vi "Scan Piezo.vi"(8 "error in (no error)":errorcluster, 9 "notifier out 2":refnum<notifier>, 10 "data":T1, 11 "Hardware Resources In":T2={"Piezo Serial Number"=41848555, "MG17Piezo"=refnum, "Setpoint (um)"=0.0}) -> (0 "error out":errorcluster, 3 "Hardware Resources Out":T2={"Piezo Serial Number"=41848555, "MG17Piezo"=refnum, "Setpoint (um)"=0.0})   [LabVIEW 2013, in "Piezo.lvlib"]
uses:
  Desktop/Simon Labview/Piezo.lvlib
  <vilib>/Platform/TimedLoop/XDataNode/wakeup.ctl
  <vilib>/Platform/TimedLoop/XDataNode/XDNodeRunTimeDep.lvlib
  <vilib>/Platform/TimedLoop/XDataNode/nitl_modes.ctl
  <vilib>/Platform/TimedLoop/XDataNode/timing_clust.ctl
  <vilib>/Platform/TimedLoop/XDataNode/XDataNode.xnode
  <vilib>/Platform/TimedLoop/scheduler/LVUserAPI/_suppVIs/Create_1kHz_TSource.vi
  Piezo State.ctl
  Hardware Configuration.ctl
  Piezo display.ctl
panel:
  in  "Scan Over":bool
  in  "Set Point":dbl
  out "Total Execution Time (s)":dbl
  out "Lag!!":bool
  in  "?":bool
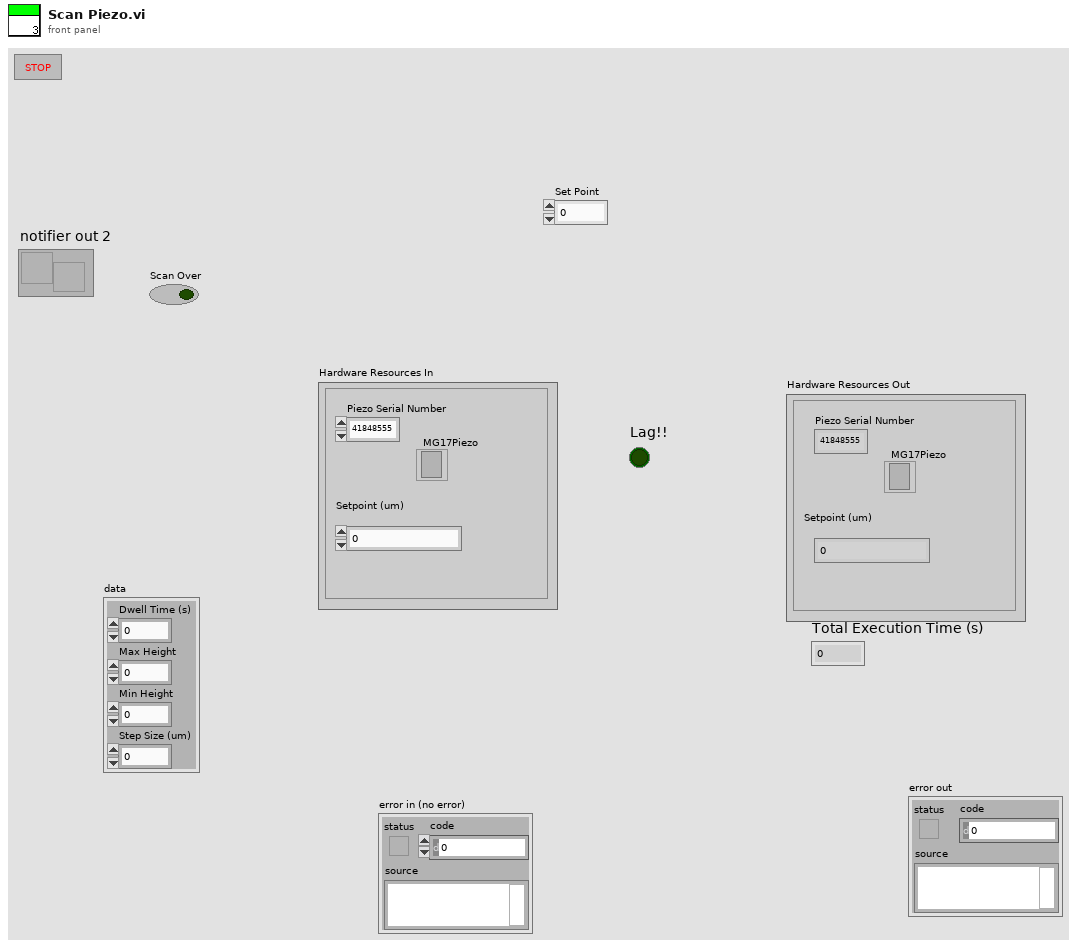
[diagram p1: front panel]
types:
  T1 = cluster{"Dwell Time (s)":dbl, "Max Height":dbl, "Min Height":dbl, "Step Size (um)":dbl}
  T2 = typedef "Piezo.lvlib/Hardware Configuration.ctl" = cluster{"Piezo Serial Number":i32, "MG17Piezo":refnum<k7>, "Setpoint (um)":sgl}
  T3 = typedef "XDNodeRunTimeDep.lvlib/timing_clust.ctl" = cluster{"Expected End [f-1]":u64, "Actual End [f-1]":u64, "Finished Late? [f-1]":bool, "Expected End [i-1]":u64, "Actual End [i-1]":u64, "Finished Late? [i-1]":bool, "Expected Start [i]":u64, "Actual Start [i]":u64, "Expected Start [f]":u64, "Actual Start [f]":u64, "Source Name":string, "Structure Name":string, "Period":i64, "Deadline":i64, "Offset":i64, "Start":i64, "Priority":i32, "Timeout":i32, "Mode":T4, "Wakeup Reason":T5, "Error":errorcluster, "Source Type":string, "Secondary Source Type":string, "Global End Time":u64, "Global Start Time":u64, "Frame Duration":u64, "Iteration Duration":u64, "Assigned CPU":i32, "I/O Scan Engine Mode":u32}
  T4 = typedef "XDNodeRunTimeDep.lvlib/nitl_modes.ctl" = enum32{"No Change", "Process missed periods, maintain original phase", "Discard missed periods, maintain original phase", "Process missed periods, ignore original phase", "Discard missed periods, ignore original phase"}
  T5 = typedef "XDNodeRunTimeDep.lvlib/wakeup.ctl" = enum32{"Normal", "Aborted", "Asynchronous wakeup", "Timing source error", "Timed loop error", "Timeout"}
  T6 = typedef "Piezo.lvlib/Piezo State.ctl" = enum16{"Idle", "Acquiring"}
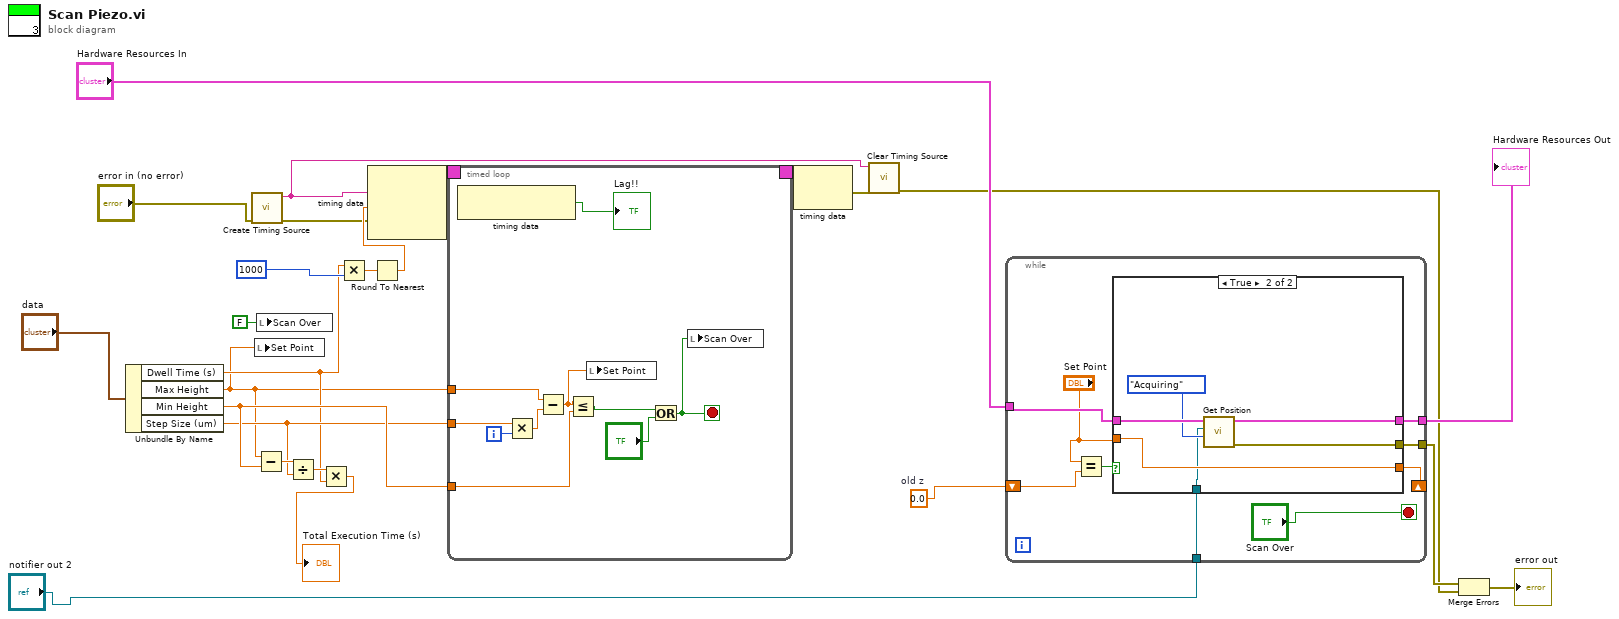
[diagram p0: block diagram]
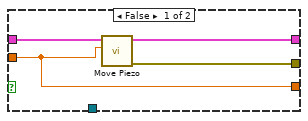
[diagram p2: hidden frame]
diagram:
  w14 = sgl 0.0  # old z
  n1 = Unbundle By Name("data") -> ("Dwell Time (s)"=w16:dbl, "Max Height"=w3:dbl, "Min Height"=w20:dbl, "Step Size (um)"=w18:dbl)
  n2 = call-poly <vilib>:"Create Timing Source.vi"("error in (no error)"="error in (no error)") -> ("error out"=w7:errorcluster, "name (out)"=w6:string)  [unwired: 9 in]
  n3 = local write "Set Point"(w3) -> ()
  n4 = Subtract(x=w3, y=w20) -> (x-y=w19:dbl)
  n5 = local write "Scan Over"(FALSE ("Scan Over")) -> ()
  n6 = Divide(x=w19, y=w18) -> (x/y=w17:dbl)
  n7 = Multiply(x=w17, y=w16) -> (x*y=→"Total Execution Time (s)":dbl)
  n8 = Multiply(x=w16, y=1000) -> (x*y=w22:dbl)
  n9 = Round To Nearest(number=w22) -> (nearest integer value=w21:dbl)
  n10 = node-c288(w6, w21, w7) -> (w25:T3)
  n11 = timed-loop {
    timing: w25 -> [_]
    timing-out: [_] -> w24
    tunnel: w18 -> [w32]
    tunnel: w20 -> [w27]
    tunnel: w3 -> [w30]
    i -> [w31]
    stop <- w29 stop-if-true
    n12 = node-c288() -> (→"Lag!!":bool)  [unwired: 1 in]
    n13 = Multiply(x=w32, y=w31) -> (x*y=w33:dbl)
    n14 = Subtract(x=w30, y=w33) -> (x-y=w26:dbl)
    n15 = Less Or Equal?(x=w26, y=w27) -> (x <= y?=w28:bool)
    n16 = local write "Set Point"(w26) -> ()
    n17 = Or(x=w28, y="?") -> (x .or. y?=w29:bool)
    n18 = local write "Scan Over"(w29) -> ()
  }
  n19 = node-c288(w24) -> (w5:errorcluster)
  n20 = call <vilib>:"Clear Timing Source.vi"("error in (no error)"=w5, "name"=w6) -> ("error out"=w4:errorcluster)  [unwired: 8 in, 1 out]
  n21 = while {
    tunnel: [w47] -> w13
    tunnel: [w46] -> w10
    tunnel: "notifier out 2" -> [w44]
    shift-right: [w43] -> _
    shift-left: w14 -> [w42]
    tunnel: "Hardware Resources In" -> [w41]
    stop <- "Scan Over" stop-if-true
    n22 = Equal?(x="Set Point", y=w42) -> (x = y?=w45:bool)
    n23 = case shown="True" w45 {
      tunnel: [w51 w57] -> w47
      tunnel: [w50 w56] -> w46
      tunnel: "Set Point" -> [w48 w55]
      tunnel: w44 -> [_ w52]
      tunnel: [w48 w55] -> w43
      tunnel: w41 -> [w49 w54]
      frame False {
        n24 = call "Move Piezo.vi"("Move to (um)"=w48, "Hardware Resources In"=w49) -> ("error out"=w50:errorcluster, "Hardware Resources Out"=w51:T2)  [unwired: 8 in]
      }
      frame True {
        n25 = call "Get Position.vi"("Hardware Resources In"=w54, "notifier out"=w52, "Piezo State"=Piezo_State."Acquiring") -> ("Hardware Resources Out"=w57:T2, "error out"=w56:errorcluster)  [unwired: 6 in]
      }
    }
  }
  "Hardware Resources Out" <- w13
  n26 = Merge Errors(w10, w4) -> (→"error out":errorcluster)
